vi "NIDMMcontTriggered.vi"() -> ()   [LabVIEW 2014]
uses:
  <instrlib>/niDMM/nidmm.llb/niDMM Sample Trigger.ctl
  <instrlib>/niDMM/nidmm.llb/niDMM ADC Calibration.ctl
  <instrlib>/niDMM/nidmm.llb/niDMM Powerline Frequency.ctl
  <instrlib>/niDMM/nidmm.llb/niDMM Configure Measurement Digits.vi
  <instrlib>/niDMM/nidmm.llb/niDMM Slope.ctl
  <instrlib>/niDMM/nidmm.llb/niDMM Trigger.ctl
  <instrlib>/niDMM/nidmm.llb/niDMM Resolution in Digits.ctl
  <instrlib>/niDMM/nidmm.llb/niDMM Function.ctl
  <instrlib>/niDMM/nidmm.llb/niDMM Measurement Complete.ctl
panel:
  in  "SlopeMeasComplete":T1 caption="Slope"
  in  "Measurement Complete Destination":T2=enum."TTL 4"
  in  "Function":T3
  in  "Resolution in Digits":T4=6.5 items=["3 1/2"=3.5, "4 1/2"=4.5, "5 1/2"=5.5, "6 1/2"=6.5, "7 1/2"=7.5]
  in  "Range":dbl=10.0 format="%.2p"
  in  "stop":bool
  out "Measurements":dbl[](graph)
  in  "Trigger Source":T5=enum."TTL 3"
  in  "Slope":T1
  in  "Device Name":refnum<k15>="PXI1Slot5"
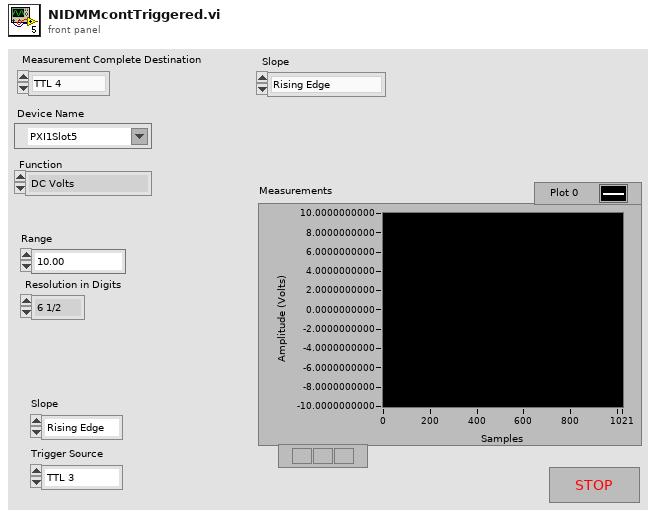
[diagram p1: front panel]
types:
  T1 = typedef "niDMM Slope.ctl" = enum16{"Rising Edge", "Falling Edge"}
  T2 = typedef "niDMM Measurement Complete.ctl" = enum16{"None", "External", "TTL 0", "TTL 1", "TTL 2", "TTL 3", "TTL 4", "TTL 5", "TTL 6", "TTL 7", "LBR Trig 0"}
  T3 = typedef "niDMM Function.ctl" = enum16{"DC Volts", "AC Volts", "DC Current", "AC Current", "2-wire Resistance", "4-wire Resistance", "Diode", "Frequency", "Period", "AC Volts DC Coupled", "Capacitance", "Inductance", "Temperature"}
  T4 = typedef "niDMM Resolution in Digits.ctl" = dbl
  T5 = typedef "niDMM Trigger.ctl" = enum16{"Immediate", "External", "TTL 0", "TTL 1", "TTL 2", "TTL 3", "TTL 4", "TTL 5", "TTL 6", "Software", "TTL 7", "PXI Star", "LBR Trig 1", "Aux Trig 1"}
  T6 = typedef "niDMM Powerline Frequency.ctl" = enum16{"60 Hz", "50 Hz"}
  T7 = typedef "niDMM ADC Calibration.ctl" = i32
  T8 = typedef "niDMM Sample Trigger.ctl" = enum16{"Immediate", "External", "TTL 0", "TTL 1", "TTL 2", "TTL 3", "TTL 4", "TTL 5", "TTL 6", "Interval", "Software", "TTL 7", "PXI Star", "LBR Trig 1", "Aux Trig 1"}
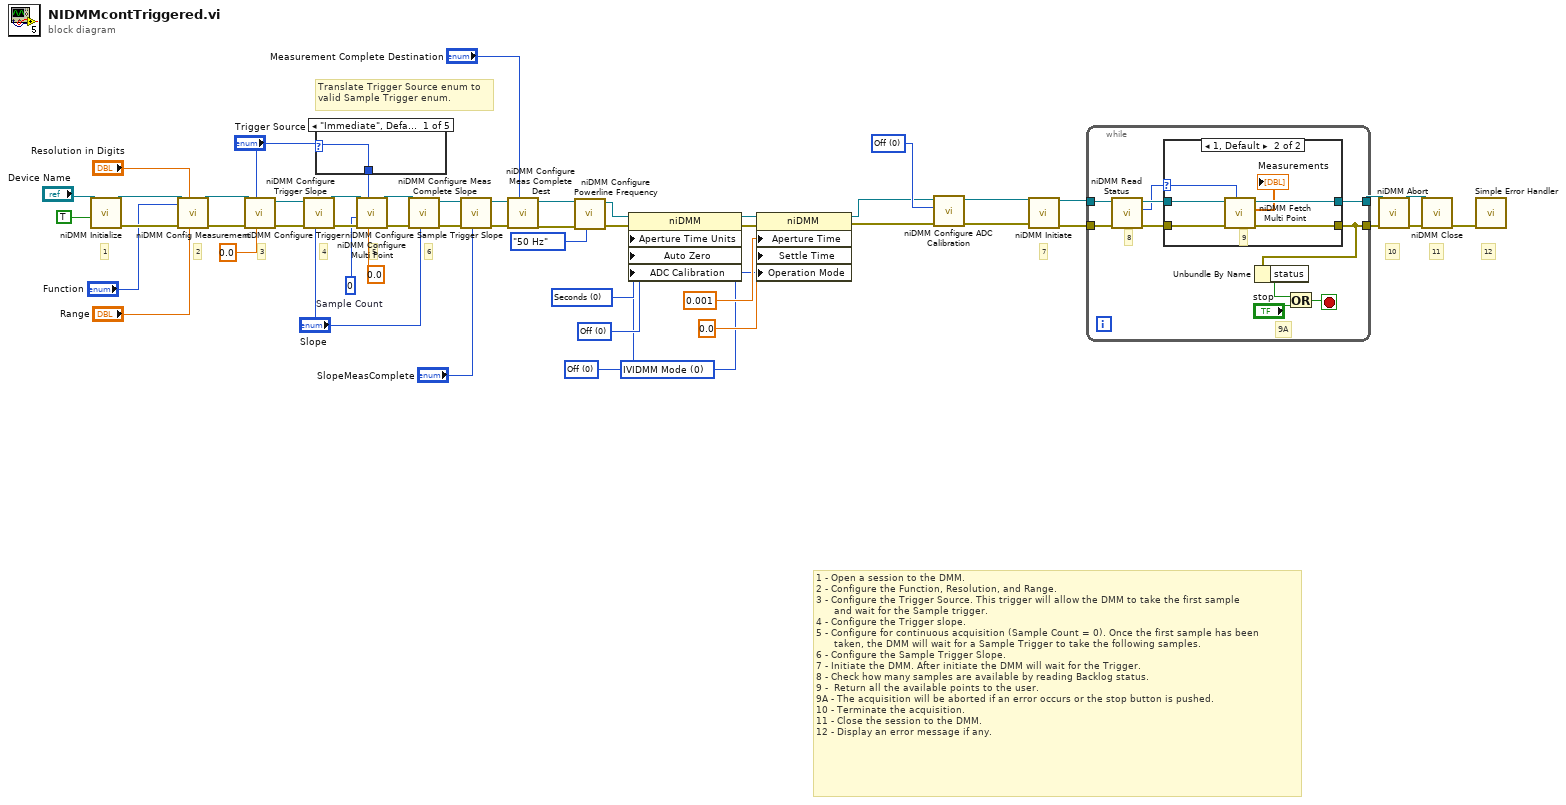
[diagram p0: block diagram]
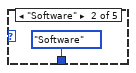
[diagram p3: hidden frame]
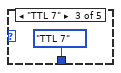
[diagram p4: hidden frame]
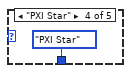
[diagram p5: hidden frame]
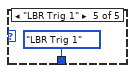
[diagram p6: hidden frame]
diagram:
  w5 = 0 items=["Auto"=-1, "Off"=0, "On"=1] ("Configuration:Measurement Options:ADC Calibration")
  w6 = 0 items=["Auto"=-1, "Off"=0, "On"=1, "Once"=2] ("Configuration:Measurement Options:Auto Zero")
  w11 = 0 items=["IVIDMM Mode", "Waveform Mode"] ("Configuration:Advanced:Operation Mode")
  w16 = 0 items=["Seconds", "Power Line Cycles"] ("Configuration:Advanced:Aperture Time Units")
  w19 = T7 0 items=["Auto"=-1, "Off"=0, "On"=1] ("ADC Calibration")
  w36 = 0  # Sample Count
  # "4"
  # "12"
  # "10"
  # "6"
  # "11"
  # "5"
  # "7"
  # "Translate Trigger Source enum to\nvalid Sample Trigger enum."
  # "3"
  # "2"
  # "1"
  # "1 - Open a session to the DMM.\n2 - Configure the Function, Resolution, and Range.\n3 - Configure the Trigger Source. This trigger will allow the DMM to take the first sample\n      and wait for the Sample trigger.\n4 - Configure the Trigger slope.\n5 - Configure for continuous acquisition (Sample Count = 0). Once the first sample has been\n      taken, the DMM will wait for a Sample Trigger to take the following samples.\n6 - Configure the Sample Trigger Slope.\n7 - Initiate the DMM. After initiate the DMM will wait for the Trigger.\n8 - Check how many samples are available by reading Backlog status.  \n9 -  Return all the available points to the user. \n9A - The acquisition will be aborted if an error occurs or the stop button is pushed.\n10 - Terminate the acquisition.\n11 - Close the session to the DMM.\n12 - Display an error message if any."
  n1 = call <instrlib>:"niDMM Initialize.vi"("Reset"=TRUE, "Instrument Descriptor"="Device Name") -> ("error out"=w51:errorcluster, "instrument handle out"=w52:refnum<k15>)  [unwired: 8 in]
  n2 = call-poly <instrlib>:"niDMM Config Measurement.vi"("Range"="Range", "Resolution in Digits"="Resolution in Digits", "error in (no error)"=w51, "Function"="Function", "instrument handle"=w52) -> ("error out"=w43:errorcluster, "instrument handle out"=w44:refnum<k15>)  [unwired: 5 in]
  n3 = call <instrlib>:"niDMM Configure Trigger.vi"("Trigger Delay (sec)"=0.0, "Trigger Source"="Trigger Source", "error in (no error)"=w43, "instrument handle"=w44) -> ("error out"=w42:errorcluster, "instrument handle out"=w17:refnum<k15>)  [unwired: 6 in]
  n4 = call <instrlib>:"niDMM Configure Trigger Slope.vi"("Slope"="Slope", "error in (no error)"=w42, "instrument handle"=w17) -> ("error out"=w40:errorcluster, "instrument handle out"=w41:refnum<k15>)  [unwired: 7 in]
  n5 = case shown="\"Immediate\", Default" "Trigger Source" {
    selector: "Trigger Source" -> [w53 _ _ _ _]
    tunnel: [w53 niDMM_Sample_Trigger."Software" ("Sample Trigger") niDMM_Sample_Trigger."TTL 7" ("Sample Trigger") niDMM_Sample_Trigger."PXI Star" ("Sample Trigger") niDMM_Sample_Trigger."LBR Trig 1" ("Sample Trigger")] -> w31
    frame "Immediate", Default {
    }
    frame "Software" {
    }
    frame "TTL 7" {
    }
    frame "PXI Star" {
    }
    frame "LBR Trig 1" {
    }
  }
  n6 = call <instrlib>:"niDMM Configure Multi Point.vi"("Sample Interval (sec)"=0.0, "Sample Trigger"=w31, "error in (no error)"=w40, "Sample Count"=w36, "instrument handle"=w41) -> ("error out"=w38:errorcluster, "instrument handle out"=w39:refnum<k15>)  [unwired: 5 in]
  n7 = call <instrlib>:"niDMM Configure Sample Trigger Slope.vi"("Slope"="Slope", "error in (no error)"=w38, "instrument handle"=w39) -> ("error out"=w24:errorcluster, "instrument handle out"=w26:refnum<k15>)  [unwired: 7 in]
  n8 = call <instrlib>:"niDMM Configure Meas Complete Slope.vi"("Slope"="SlopeMeasComplete", "error in (no error)"=w24, "instrument handle"=w26) -> ("error out"=w23:errorcluster, "instrument handle out"=w25:refnum<k15>)  [unwired: 7 in]
  n9 = call <instrlib>:"niDMM Configure Meas Complete Dest.vi"("Measurement Complete Destination"="Measurement Complete Destination", "error in (no error)"=w23, "instrument handle"=w25) -> ("error out"=w4:errorcluster, "instrument handle out"=w3:refnum<k15>)  [unwired: 7 in]
  n10 = call <instrlib>:"niDMM Configure Powerline Frequency.vi"("Powerline Frequency"=niDMM_Powerline_Frequency."50 Hz", "error in (no error)"=w4, "instrument handle"=w3) -> ("error out"=w1:errorcluster, "instrument handle out"=w2:refnum<k15>)  [unwired: 7 in]
  n11 = property class="niDMM"(reference=w2, error in=w1, "Aperture Time Units"=w16, "Auto Zero"=w6, "ADC Calibration"=w5) -> (reference out=w15:refnum<k15>, error out=w14:errorcluster)
  n12 = property class="niDMM"(reference=w15, error in=w14, "Aperture Time"=0.001 ("Configuration:Advanced:Aperture Time"), "Settle Time"=0.0 ("Configuration:Advanced:Settle Time"), "Operation Mode"=w11) -> (reference out=w10:refnum<k15>, error out=w9:errorcluster)
  n13 = call <instrlib>:"niDMM Configure ADC Calibration.vi"("error in (no error)"=w9, "ADC Calibration"=w19, "instrument handle"=w10) -> ("error out"=w8:errorcluster, "instrument handle out"=w7:refnum<k15>)  [unwired: 7 in]
  n14 = call <instrlib>:"niDMM Initiate.vi"("error in (no error)"=w8, "instrument handle"=w7) -> ("error out"=w50:errorcluster, "instrument handle out"=w49:refnum<k15>)  [unwired: 8 in]
  n15 = while {
    tunnel: [w67] -> w33
    tunnel: w49 -> [w63]
    tunnel: [w59] -> w34
    tunnel: w50 -> [w62]
    stop <- w64 stop-if-true
    # "9A"
    # "8"
    n16 = call <instrlib>:"niDMM Read Status.vi"("error in (no error)"=w62, "instrument handle"=w63) -> ("error out"=w61:errorcluster, "Backlog"=w58:i32, "instrument handle out"=w60:refnum<k15>)  [unwired: 6 in, 1 out]
    n17 = case shown="1, Default" w58 {
      selector: w58 -> [_ w70]
      tunnel: [w69 w75] -> w67
      tunnel: [w68 w73] -> w59
      tunnel: w61 -> [w68 w72]
      tunnel: w60 -> [w69 w71]
      frame 0 {
      }
      frame 1, Default {
        # "9"
        n18 = call <instrlib>:"niDMM Fetch Multi Point.vi"("Number to Fetch"=w70, "error in (no error)"=w72, "instrument handle"=w71) -> ("error out"=w73:errorcluster, "Measurements"=→"Measurements":dbl[], "instrument handle out"=w75:refnum<k15>)  [unwired: 5 in, 1 out]
      }
    }
    n19 = Unbundle By Name(w59) -> ("status"=w66:bool)
    n20 = Or(x=w66, y="stop") -> (x .or. y?=w64:bool)
  }
  n21 = call <instrlib>:"niDMM Abort.vi"("error in (no error)"=w34, "instrument handle"=w33) -> ("error out"=w47:errorcluster, "instrument handle out"=w48:refnum<k15>)  [unwired: 8 in]
  n22 = call <instrlib>:"niDMM Close.vi"("error in (no error)"=w47, "instrument handle"=w48) -> ("error out"=w30:errorcluster)  [unwired: 9 in]
  n23 = call <vilib>:"Simple Error Handler.vi"("error in (no error)"=w30) -> ()  [unwired: 4 in, 5 out]
